vi "KH TURCK ETHERNETIP IOL Diagnostic Bits.vi"(8 "Bit Offset":i32=4, 10 "Start Byte":i32=4, 11 "DataItem.Data":u8[](array[numeric])) -> (0 "Bit D":bool, 1 "Bit C":bool, 2 "Bit B":bool, 3 "Bit A":bool)   [LabVIEW 2021]
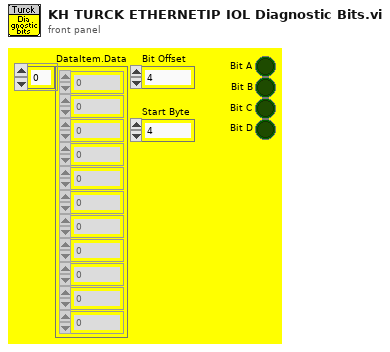
[diagram p1: front panel]
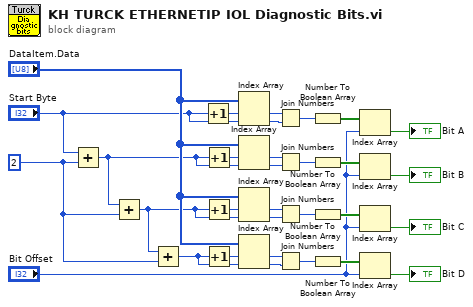
[diagram p0: block diagram]
diagram:
  w21 = 2 ("y")
  n1 = Add(x="Start Byte", y=w21) -> (x+y=w5:i32)
  n2 = Add(x=w5, y=w21) -> (x+y=w3:i32)
  n3 = Add(x=w3, y=w21) -> (x+y=w1:i32)
  n4 = Increment(x="Start Byte") -> (x+1=w8:i32)
  n5 = Increment(x=w5) -> (x+1=w6:i32)
  n6 = Increment(x=w3) -> (x+1=w4:i32)
  n7 = Increment(x=w1) -> (x+1=w2:i32)
  n8 = Index Array(array="DataItem.Data", index #1=w8, index #2="Start Byte") -> (element #1=w20:u8, element #2=w19:u8)
  n9 = Index Array(array="DataItem.Data", index #1=w6, index #2=w5) -> (element #1=w17:u8, element #2=w16:u8)
  n10 = Index Array(array="DataItem.Data", index #1=w4, index #2=w3) -> (element #1=w15:u8, element #2=w14:u8)
  n11 = Index Array(array="DataItem.Data", index #1=w2, index #2=w1) -> (element #1=w13:u8, element #2=w12:u8)
  n12 = Join Numbers(hi=w20, lo=w19) -> ((hi.lo)=w18:u16)
  n13 = Join Numbers(hi=w17, lo=w16) -> ((hi.lo)=w10:u16)
  n14 = Join Numbers(hi=w15, lo=w14) -> ((hi.lo)=w9:u16)
  n15 = Join Numbers(hi=w13, lo=w12) -> ((hi.lo)=w11:u16)
  n16 = Number To Boolean Array(number=w18) -> (Boolean array=w28:bool[])
  n17 = Number To Boolean Array(number=w10) -> (Boolean array=w29:bool[])
  n18 = Number To Boolean Array(number=w9) -> (Boolean array=w30:bool[])
  n19 = Number To Boolean Array(number=w11) -> (Boolean array=w31:bool[])
  n20 = Index Array(array=w28, index="Bit Offset") -> (element=→"Bit A":bool)
  n21 = Index Array(array=w29, index="Bit Offset") -> (element=→"Bit B":bool)
  n22 = Index Array(array=w30, index="Bit Offset") -> (element=→"Bit C":bool)
  n23 = Index Array(array=w31, index="Bit Offset") -> (element=→"Bit D":bool)
